vi "listcolumns.vi"(8 "error in (no error)":errorcluster caption="错误输入（无错误）", 10 "table":string, 11 "access 输入":refnum<class "access.lvclass">) -> (0 "error out":errorcluster caption="错误输出", 2 "columns":string[](array[string]), 3 "access 输出":refnum<class "access.lvclass">)   [LabVIEW 2016, in "中水三立SQL数据传输.lvlib" / "access.lvclass"]
uses:
  access.lvclass
  <vilib>/addons/database/NI_Database_API.lvlib
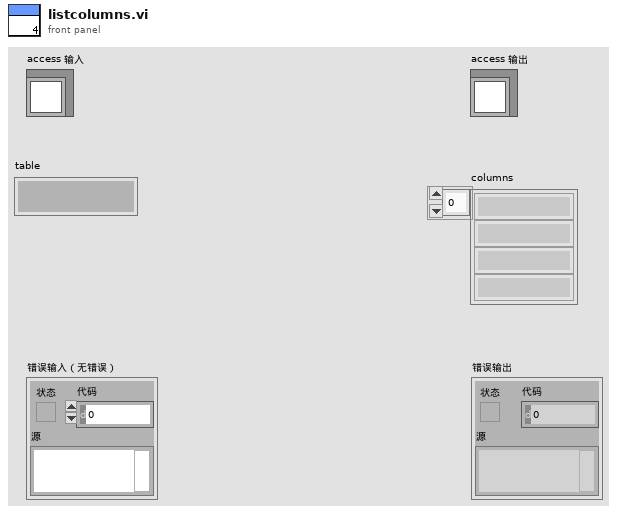
[diagram p1: front panel]
types:
  T1 = typedef "NI_Database_API.lvlib/Conn ObjectReference.ctl" = refnum<k1>
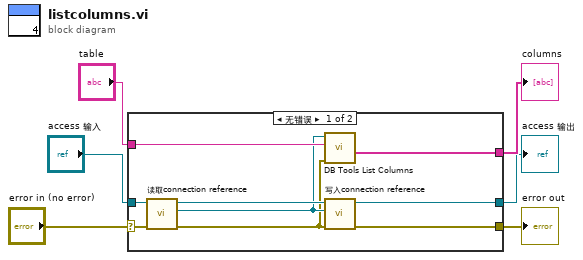
[diagram p0: block diagram]
diagram:
  n1 = case shown="无错误" "error in (no error)" {
    selector: "error in (no error)" -> [w9 w17]
    tunnel: "table" -> [w15 _]
    tunnel: "access 输入" -> [w13 w16]
    tunnel: [w14 _] -> w4
    tunnel: [w11 w16] -> w3
    tunnel: [w10 w17] -> w2
    frame No Error {
      n2 = call-dynamic "读取connection reference.vi"("error in (no error)"=w9, "database输入"=w13) -> ("error out"=w7:errorcluster, "reference"=w8:T1, "database输出"=w12:refnum<class "access.lvclass">)  [unwired: 7 in]
      n3 = call <vilib>:"DB Tools List Columns.vi"("error in (no error)"=w7, "table"=w15, "connection reference"=w8) -> ("columns"=w14:string[])  [unwired: 1 in, 3 out]
      n4 = call-dynamic "写入connection reference.vi"("error in (no error)"=w7, "reference"=w8, "database输入"=w12) -> ("error out"=w10:errorcluster, "database输出"=w11:refnum<class "access.lvclass">)  [unwired: 7 in]
    }
    frame Error {
    }
  }
  "error out" <- w2
  "access 输出" <- w3
  "columns" <- w4
